vi "Labview7.vi"() -> ()   [LabVIEW 2016]
panel:
  in  "stop":bool
  in  "Keep Previous Locations":bool
  out "2D Picture":picture
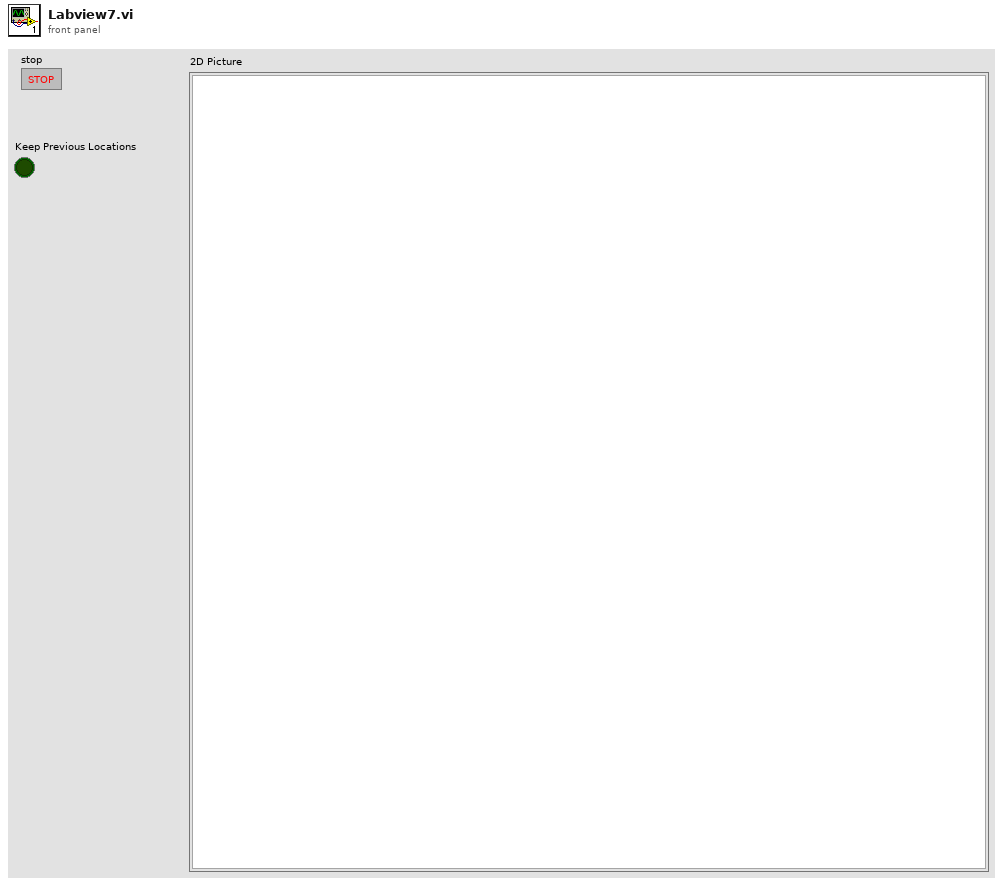
[diagram p1: front panel]
types:
  T1 = cluster{"Width":u16, "Style":enum32{"Solid", "Dash", "Dot", "DashDot", "DashDotDot"}}
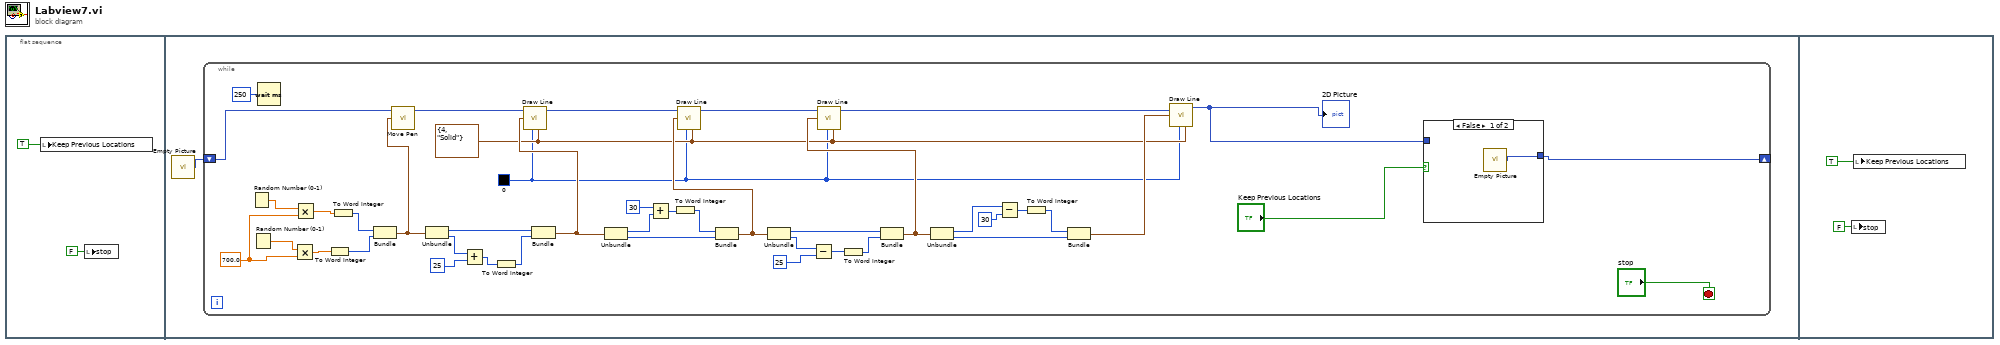
[diagram p0: block diagram]
diagram:
  n1 = flat-sequence {
    frame #0 {
      n2 = local write "Keep Previous Locations"(TRUE ("Keep Previous Locations")) -> ()
      n3 = local write "stop"(FALSE ("stop")) -> ()
    }
    frame #1 {
      n4 = call "Empty Picture"() -> ("empty picture"=w3:picture)
      n5 = while {
        shift-right: [w6] -> _
        shift-left: w3 -> [w44]
        stop <- "stop" stop-if-true
        w4 = u32 0 ("color(black)")
        w7 = T1 {"Width"=4, "Style"=enum."Solid"} ("pen")
        w37 = 700.0 ("y")
        n6 = Random Number (0-1)() -> (number: 0 to 1=w39:dbl)
        n7 = Random Number (0-1)() -> (number: 0 to 1=w38:dbl)
        n8 = Wait (ms)(milliseconds to wait=u32 250) -> ()  [unwired: 1 out]
        n9 = Multiply(x=w38, y=w37) -> (x*y=w36:dbl)
        n10 = Multiply(x=w39, y=w37) -> (x*y=w35:dbl)
        n11 = To Word Integer(number=w36) -> (16bit integer=w33:i16)
        n12 = To Word Integer(number=w35) -> (16bit integer=w34:i16)
        n13 = Bundle(w34, w33) -> (w32:cluster{i16, i16})  [unwired: 1 in]
        n14 = call <vilib>:"Move Pen.vi"("new position"=w32, "picture"=w44) -> ("new picture"=w43:picture)  [unwired: 3 in]
        n15 = Unbundle(w32) -> (w31:i16, w30:i16)
        n16 = Add(x=w30, y=i16 25) -> (x+y=w28:i16)
        n17 = To Word Integer(number=w28) -> (16bit integer=w27:i16)
        n18 = Bundle(w31, w27) -> (w26:cluster{i16, i16})  [unwired: 1 in]
        n19 = call <vilib>:"Draw Line.vi"("picture"=w43, "end point"=w26, "color(black)"=w4, "pen"=w7) -> ("new picture"=w42:picture)  [unwired: 5 in]
        n20 = Unbundle(w26) -> (w24:i16, w25:i16)
        n21 = Add(x=i16 30, y=w24) -> (x+y=w22:i16)
        n22 = To Word Integer(number=w22) -> (16bit integer=w21:i16)
        n23 = Bundle(w21, w25) -> (w20:cluster{i16, i16})  [unwired: 1 in]
        n24 = call <vilib>:"Draw Line.vi"("picture"=w42, "end point"=w20, "color(black)"=w4, "pen"=w7) -> ("new picture"=w41:picture)  [unwired: 5 in]
        n25 = Unbundle(w20) -> (w19:i16, w18:i16)
        n26 = Subtract(x=w18, y=i16 25) -> (x-y=w16:i16)
        n27 = To Word Integer(number=w16) -> (16bit integer=w15:i16)
        n28 = Bundle(w19, w15) -> (w14:cluster{i16, i16})  [unwired: 1 in]
        n29 = call <vilib>:"Draw Line.vi"("picture"=w41, "end point"=w14, "color(black)"=w4, "pen"=w7) -> ("new picture"=w40:picture)  [unwired: 5 in]
        n30 = Unbundle(w14) -> (w12:i16, w13:i16)
        n31 = Subtract(x=w12, y=i16 30) -> (x-y=w10:i16)
        n32 = To Word Integer(number=w10) -> (16bit integer=w9:i16)
        n33 = Bundle(w9, w13) -> (w8:cluster{i16, i16})  [unwired: 1 in]
        n34 = call <vilib>:"Draw Line.vi"("picture"=w40, "end point"=w8, "color(black)"=w4, "pen"=w7) -> ("new picture"=w5:picture)  [unwired: 5 in]
        "2D Picture" <- w5
        n35 = case shown="False" "Keep Previous Locations" {
          tunnel: [w48 w49] -> w6
          tunnel: w5 -> [_ w49]
          frame False {
            n36 = call "Empty Picture"() -> ("empty picture"=w48:picture)
          }
          frame True {
          }
        }
      }
    }
    frame #2 {
      n37 = local write "stop"(FALSE ("stop")) -> ()
      n38 = local write "Keep Previous Locations"(TRUE ("Keep Previous Locations")) -> ()
    }
  }
